vi "PH_PILS.Dialog Enabling PW.vi"() -> (16 "User Name":string, 18 "o.k.":bool)   [LabVIEW 2014, in "PH_PILS.lvlib"]
doc: "This VI containes the Dialog for the enabling procedure. The User has to enter his/her password."
uses:
  PH_PILS.lvlib
panel:
  in  "Cancel Button":bool
  in  "Please enter your password:":string
  in  "OK Button":bool
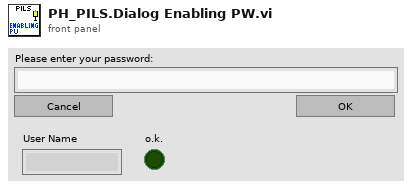
[diagram p1: front panel]
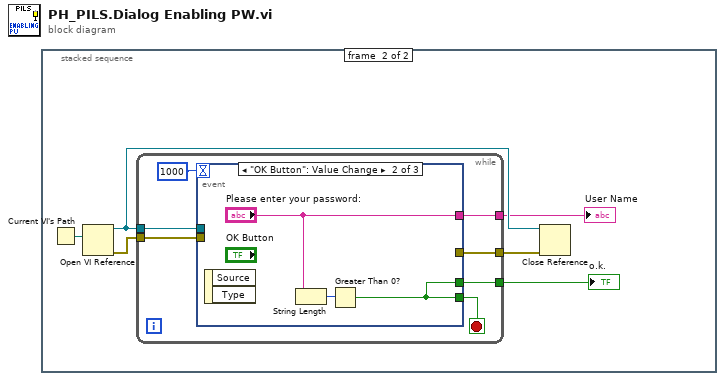
[diagram p0: block diagram]
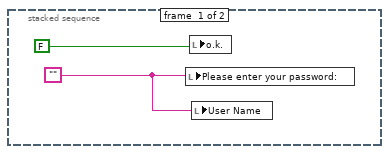
[diagram p2: hidden frame]
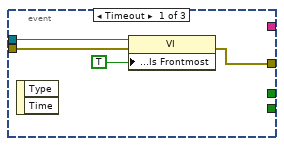
[diagram p3: hidden frame]
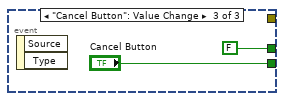
[diagram p4: hidden frame]
diagram:
  n1 = stacked-sequence {
    frame #0 {
      w1 = ""
      n2 = local write "Please enter your password:"(w1) -> ()
      n3 = local write "o.k."(FALSE) -> ()
      n4 = local write "User Name"(w1) -> ()
    }
    frame #1 {
      n5 = Current VI's Path() -> (path=w8:path)
      n6 = Open VI Reference(vi path=w8) -> (vi reference=w5:refnum<vi>, error out=w7:errorcluster)  [unwired: 5 in]
      n7 = while {
        tunnel: [w15] -> w4
        tunnel: w5 -> [w13]
        tunnel: w7 -> [w12]
        tunnel: [w11] -> w6
        tunnel: [w9] -> w3
        stop <- w10 stop-if-true
        n8 = event shown="[1] \"OK Button\": Value Change" {
          selector: _ -> [_ _ _]
          dyn-events: _ -> [_ _ _]
          timeout: 1000 -> [_ _ _]
          tunnel: [_ w20 "Cancel Button"] -> w10
          tunnel: [_ "Please enter your password:" _] -> w15
          tunnel: w13 -> [w19 _ _]
          tunnel: w12 -> [w18 _ _]
          tunnel: [w16 _ _] -> w11
          tunnel: [_ w20 FALSE] -> w9
          event Timeout {
            n9 = event-data() -> ()  [unwired: 1 in, 2 out]
            n10 = property class="VI"(reference=w19, error in=w18, "Front Panel Window:Is Frontmost"=TRUE) -> (error out=w16:errorcluster)  [unwired: 1 out]
          }
          event "OK Button": Value Change {
            n11 = event-data() -> ()  [unwired: 1 in, 2 out]
            n12 = String Length(string="Please enter your password:") -> (length=w22:i32)
            n13 = Greater Than 0?(x=w22) -> (x > 0?=w20:bool)
          }
          event "Cancel Button": Value Change {
            n14 = event-data() -> ()  [unwired: 1 in, 2 out]
          }
        }
      }
      "User Name" <- w4
      "o.k." <- w3
      n15 = Close Reference(reference=w5, error in (no error)=w6) -> ()  [unwired: 1 out]
    }
  }
